vi "Combine_Anomaly_Detection_Results.vi"(4 "Infrnc Dims":cluster{"X Resolution":i32, "Y Resolution":i32}={"X Resolution"=224, "Y Resolution"=224}, 5 "Pixel Results":T1={"Scores(Good)"={"Min"=4.5729, "Max"=58.2981}, "Scores(Bad)"={"Min"=22.3012, "Max"=57.8689}, "F1_Max"=0.3453, "Thrshld(F1_Max)"=38.5075, "IoU_Max"=0.2087, "Thrshld(IoU_Max)"=38.5075, "AUROC"=0.9874, "Prec.(F1_Max)"=0.3041, "Recall(F1_Max)"=0.3994, "FPR(F1_Max)"=0.6006, "FNR(F1_Max)"=0.0} {"FPR(F1_Max)" format="%#_5g"; "FNR(F1_Max)" format="%#_5g"; "Scores(Bad)"."Min" format="%#_5g"; "Scores(Good)"."Min" format="%#_5g"}, 6 "Heatmap Config":T3={"ColorMap_Type"=enum."Jet", "Alpha"=0.4, "Heatmap Range"={"Min"=-1.0, "Max"=-1.0}} {"Heatmap Range"."Min" format="%#_5g"}, 7 "Pixel Anomaly Thrshld":sgl=60.0 format="%_4g", 8 "error in":errorcluster, 9 "Anomaly Map":sgl[][](array[numeric]), 10 "Gt File Path":path, 11 "Img File Path":path=path "D:/DNN/MVTec/screw/test/scratch_head/015.png") -> (0 "error out":errorcluster, 2 "Actual Pixel Threshold":sgl=60.0, 3 "Anomaly Detection Rresults":T5={"Image"="remote image 000001EE05A87998", "Ground Truth"="remote image 000001EE05A87DB8", "Predicted Heat Map"="remote image 000001EE05A87F18", "Predicted Mask"="remote image 000001EE05A87FC8", "Segmentation"="remote image 000001EE05A88968"})   [LabVIEW 2020]
uses:
  PatchCore_AddOn/Low_Level/Controls/Anomaly_Detection_Results_Imgs.ctl
  PatchCore_AddOn/API/Controls/Heatmap_Config.ctl
  PatchCore_AddOn/API/Controls/ColorMap.ctl
  PatchCore_AddOn/API/Controls/MinMax.ctl
  PatchCore_AddOn/API/Controls/Eval_Results.ctl
  <vilib>/vision/Image Controls.llb/IMAQ Image.ctl
  <vilib>/vision/NI_Vision_Development_Module.lvlib
  PatchCore_AddOn/PatchCore_AddOn.lvlib
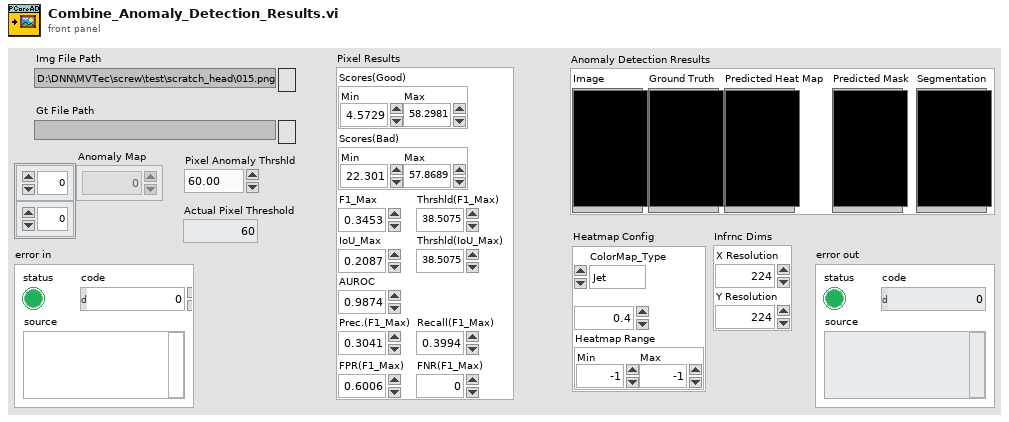
[diagram p1: front panel]
types:
  T1 = typedef "PatchCore_AddOn.lvlib/Eval_Results.ctl" = cluster{"Scores(Good)":T2, "Scores(Bad)":T2, "F1_Max":sgl, "Thrshld(F1_Max)":sgl, "IoU_Max":sgl, "Thrshld(IoU_Max)":sgl, "AUROC":sgl, "Prec.(F1_Max)":sgl, "Recall(F1_Max)":sgl, "FPR(F1_Max)":sgl, "FNR(F1_Max)":sgl}
  T2 = typedef "PatchCore_AddOn.lvlib/MinMax.ctl" = cluster{"Min":sgl, "Max":sgl}
  T3 = typedef "PatchCore_AddOn.lvlib/Heatmap_Config.ctl" = cluster{"ColorMap_Type":T4, "Alpha":sgl, "Heatmap Range":T2}
  T4 = typedef "PatchCore_AddOn.lvlib/ColorMap.ctl" = enum16{"Jet", "Perula", "Inferno", "Plasma", "Viridis"}
  T5 = typedef "PatchCore_AddOn.lvlib/Anomaly_Detection_Results_Imgs.ctl" = cluster{"Image":T6, "Ground Truth":T6, "Predicted Heat Map":T6, "Predicted Mask":T6, "Segmentation":T6}
  T6 = typedef "IMAQ Image.ctl" = refnum<image>
  T7 = typedef "Image Type" = u32
  T8 = cluster{"X Resolution":bool, "Y Resolution":bool}
  T9 = typedef "ROI Descriptor" = cluster{"Global Rectangle":i32[], "Contours":cluster{"ID":enum32{"External", "Internal"}, "Type":u32, "Coordinates":i32[]}[]}
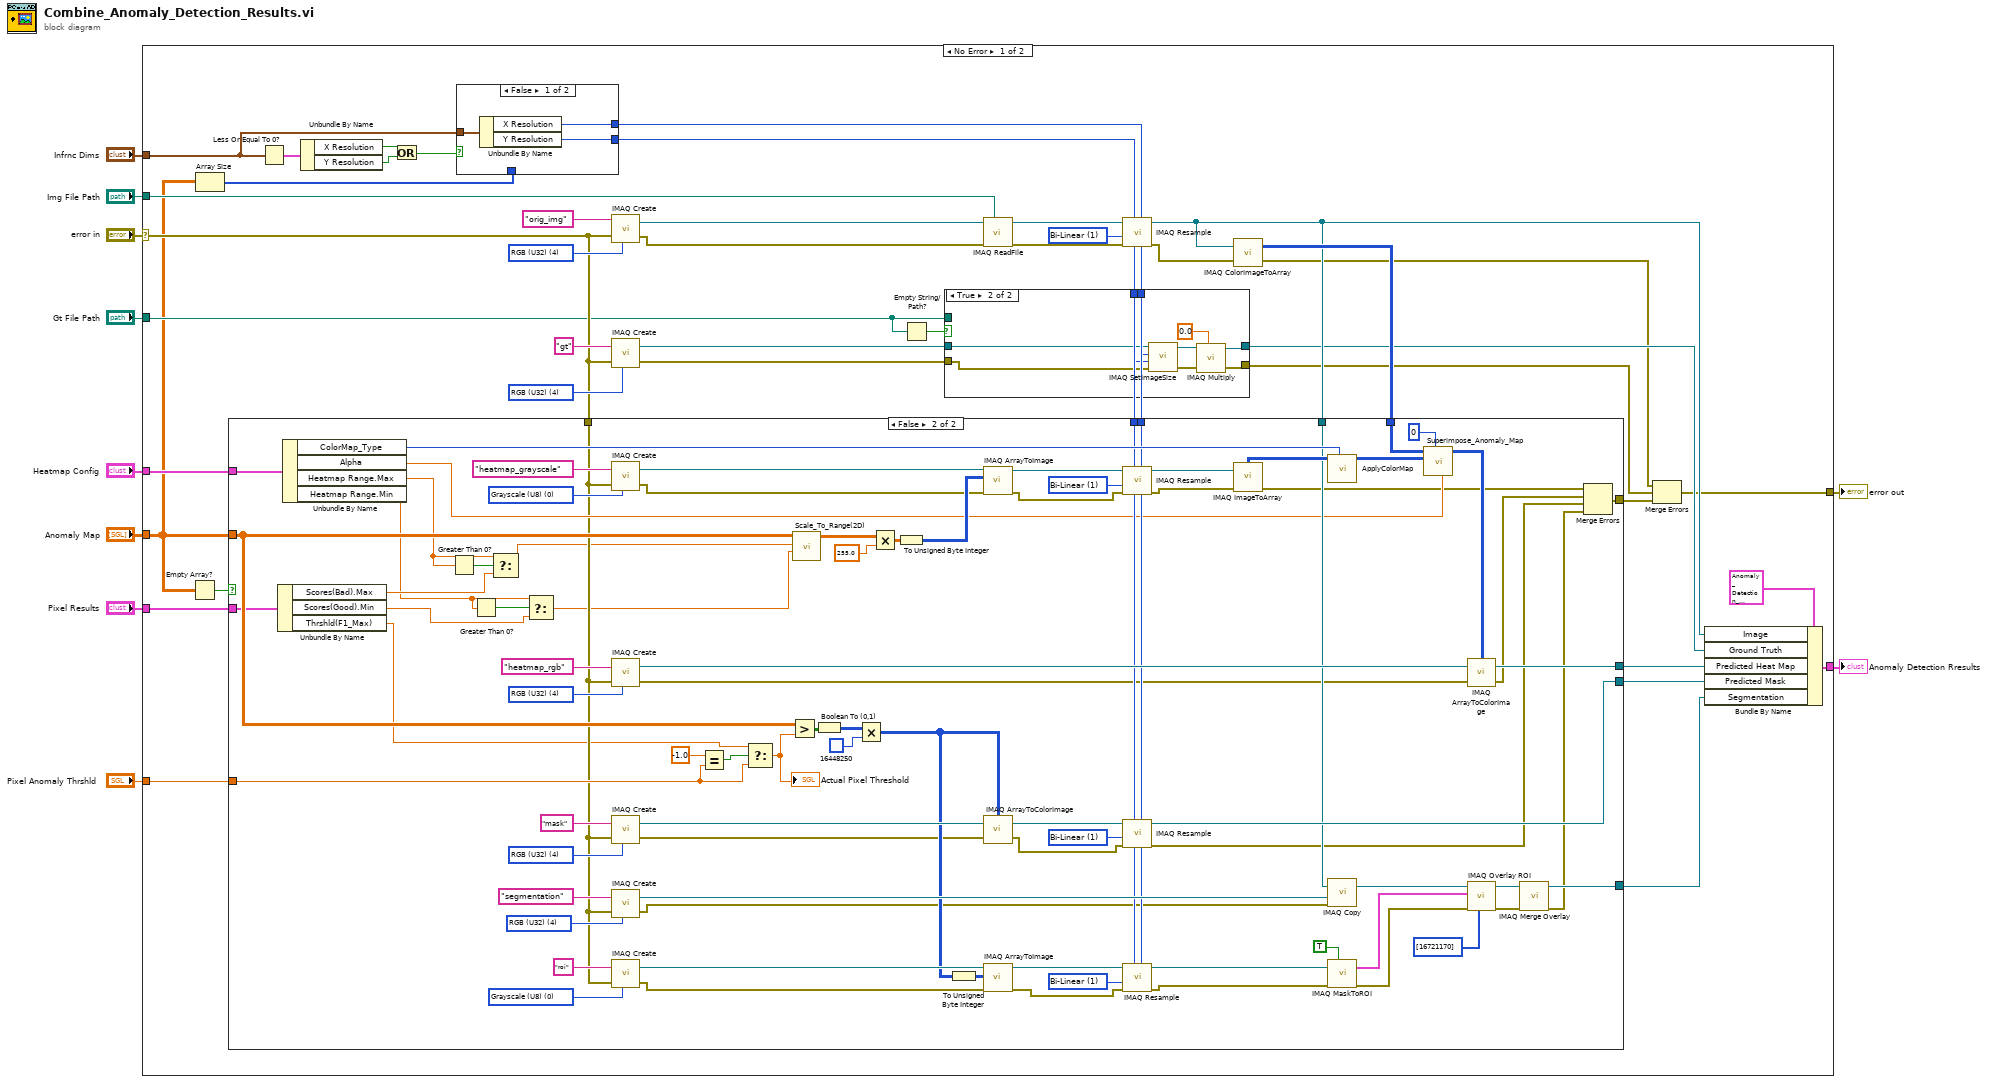
[diagram p0: block diagram]
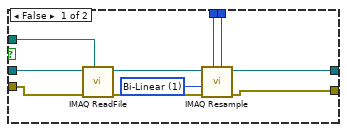
[diagram p3: hidden frame]
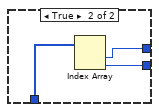
[diagram p4: hidden frame]
diagram:
  n1 = case shown="No Error" "error in" {
    selector: "error in" -> [w19 w162]
    tunnel: [w47 _] -> w10
    tunnel: "Heatmap Config" -> [w43 _]
    tunnel: "Img File Path" -> [w40 _]
    tunnel: "Pixel Anomaly Thrshld" -> [w38 _]
    tunnel: "Infrnc Dims" -> [w29 _]
    tunnel: "Pixel Results" -> [w27 _]
    tunnel: "Gt File Path" -> [w18 _]
    tunnel: [w13 w162] -> w2
    tunnel: "Anomaly Map" -> [w12 _]
    frame No Error {
      w22 = u32 1 items=["Zero Order", "Bi-Linear", "Quadratic", "Cubic Spline"] ("Interpolation Type")
      w39 = T7 4 items=["Grayscale (U8)", "Grayscale (I16)", "Grayscale (SGL)", "Complex (CSG)", "RGB (U32)", "HSL (U32)", "RGB (U64)", "Grayscale (U16)"] ("Image Type")
      w50 = T7 4 items=["Grayscale (U8)", "Grayscale (I16)", "Grayscale (SGL)", "Complex (CSG)", "RGB (U32)", "HSL (U32)", "RGB (U64)", "Grayscale (U16)"] ("Image Type")
      n2 = Empty Array?(array=w12) -> (empty?=w11:bool)
      n3 = Array Size(array=w12) -> (size(s)=w28:i32[])
      n4 = Less Or Equal To 0?(x=w29) -> (x <= 0?=w33:T8)
      n5 = Unbundle By Name(w33) -> ("X Resolution"=w32:bool, "Y Resolution"=w31:bool)
      n6 = Or(x=w32, y=w31) -> (x .or. y?=w30:bool)
      n7 = case shown="False" w30 {
        tunnel: w29 -> [w158 _]
        tunnel: [w157 w160] -> w24
        tunnel: [w156 w159] -> w23
        tunnel: w28 -> [_ w161]
        frame False {
          n8 = Unbundle By Name(w158) -> ("X Resolution"=w157:i32, "Y Resolution"=w156:i32)
        }
        frame True {
          n9 = Index Array(array=w161) -> (element #1=w160:i32, element #2=w159:i32)  [unwired: 2 in]
        }
      }
      n10 = call "IMAQ Create"("Image Name"="orig_img", "Image Type"=w39, "error in (no error)"=w19) -> ("New Image"=w41:T6, "error out"=w20:errorcluster)  [unwired: 2 in]
      n11 = call "IMAQ Create"("Image Name"="gt", "Image Type"=w50, "error in (no error)"=w19) -> ("New Image"=w25:T6, "error out"=w17:errorcluster)  [unwired: 2 in]
      n12 = Empty String/Path?(string/path=w18) -> (empty?=w26:bool)
      n13 = case shown="True" w26 {
        tunnel: w25 -> [w146 w155]
        tunnel: w18 -> [w145 _]
        tunnel: [w144 w149] -> w34
        tunnel: [w142 w148] -> w15
        tunnel: w24 -> [w140 w154]
        tunnel: w23 -> [w139 w153]
        tunnel: w17 -> [w137 w147]
        frame False {
          w138 = u32 1 items=["Zero Order", "Bi-Linear", "Quadratic", "Cubic Spline"] ("Interpolation Type")
          n14 = call "IMAQ ReadFile"("File Path"=w145, "error in (no error)"=w137, "Image"=w146) -> ("error out"=w143:errorcluster, "Image Out"=w141:T6)  [unwired: 4 in, 3 out]
          n15 = call "IMAQ Resample"("X Resolution"=w140, "Y Resolution"=w139, "error in (no error)"=w143, "Interpolation Type"=w138, "Image Src"=w141) -> ("error out"=w142:errorcluster, "Image Dst Out"=w144:T6)  [unwired: 5 in]
        }
        frame True {
          n16 = call "IMAQ SetImageSize"("error in (no error)"=w147, "Y Resolution"=w153, "X Resolution"=w154, "Image"=w155) -> ("error out"=w152:errorcluster, "Image Out"=w151:T6)  [unwired: 1 in]
          n17 = call "IMAQ Multiply"("Image Src A"=w151, "Constant"=0.0, "error in (no error)"=w152) -> ("Image Dst Out"=w149:T6, "error out"=w148:errorcluster)  [unwired: 4 in]
        }
      }
      n18 = call "IMAQ ReadFile"("File Path"=w40, "error in (no error)"=w20, "Image"=w41) -> ("error out"=w35:errorcluster, "Image Out"=w36:T6)  [unwired: 4 in, 3 out]
      n19 = call "IMAQ Resample"("X Resolution"=w24, "Y Resolution"=w23, "error in (no error)"=w35, "Interpolation Type"=w22, "Image Src"=w36) -> ("error out"=w21:errorcluster, "Image Dst Out"=w37:T6)  [unwired: 5 in]
      n20 = call "IMAQ ColorImageToArray"("Image"=w37, "error in (no error)"=w21) -> ("Image Pixels (U32)"=w48:u32[][], "error out"=w16:errorcluster)  [unwired: 2 in, 1 out]
      n21 = case shown="False" w11 {
        tunnel: w48 -> [_ w119]
        tunnel: [_ w107] -> w46
        tunnel: [_ w105] -> w45
        tunnel: [_ w104] -> w44
        tunnel: w43 -> [_ w90]
        tunnel: w38 -> [_ w88]
        tunnel: w37 -> [_ w84]
        tunnel: w12 -> [_ w81]
        tunnel: w27 -> [_ w80]
        tunnel: w24 -> [_ w78]
        tunnel: w23 -> [_ w77]
        tunnel: w19 -> [w52 w74]
        tunnel: [w52 w62] -> w14
        frame True {
        }
        frame False {
          w82 = u32 1 items=["Zero Order", "Bi-Linear", "Quadratic", "Cubic Spline"] ("Interpolation Type")
          w96 = u32 1 items=["Zero Order", "Bi-Linear", "Quadratic", "Cubic Spline"] ("Interpolation Type")
          w100 = T7 0 items=["Grayscale (U8)", "Grayscale (I16)", "Grayscale (SGL)", "Complex (CSG)", "RGB (U32)", "HSL (U32)", "RGB (U64)", "Grayscale (U16)"] ("Image Type")
          w112 = u32 1 items=["Zero Order", "Bi-Linear", "Quadratic", "Cubic Spline"] ("Interpolation Type")
          w117 = T7 4 items=["Grayscale (U8)", "Grayscale (I16)", "Grayscale (SGL)", "Complex (CSG)", "RGB (U32)", "HSL (U32)", "RGB (U64)", "Grayscale (U16)"] ("Image Type")
          w122 = T7 4 items=["Grayscale (U8)", "Grayscale (I16)", "Grayscale (SGL)", "Complex (CSG)", "RGB (U32)", "HSL (U32)", "RGB (U64)", "Grayscale (U16)"] ("Image Type")
          w125 = T7 4 items=["Grayscale (U8)", "Grayscale (I16)", "Grayscale (SGL)", "Complex (CSG)", "RGB (U32)", "HSL (U32)", "RGB (U64)", "Grayscale (U16)"] ("Image Type")
          w135 = T7 0 items=["Grayscale (U8)", "Grayscale (I16)", "Grayscale (SGL)", "Complex (CSG)", "RGB (U32)", "HSL (U32)", "RGB (U64)", "Grayscale (U16)"] ("Image Type")
          n22 = Unbundle By Name(w80) -> ("Scores(Bad).Max"=w60:sgl, "Scores(Good).Min"=w57:sgl, "Thrshld(F1_Max)"=w55:sgl)
          n23 = Unbundle By Name(w90) -> ("ColorMap_Type"=w89:T4, "Alpha"=w76:sgl, "Heatmap Range.Max"=w53:sgl, "Heatmap Range.Min"=w54:sgl)
          n24 = Greater Than 0?(x=w53) -> (x > 0?=w59:bool)
          n25 = Greater Than 0?(x=w54) -> (x > 0?=w56:bool)
          n26 = Select(t=w53, s=w59, f=w60) -> (s? t:f=w61:sgl)
          n27 = Select(t=w54, s=w56, f=w57) -> (s? t:f=w58:sgl)
          n28 = call "IMAQ Create"("Image Name"="heatmap_grayscale", "Image Type"=w100, "error in (no error)"=w74) -> ("New Image"=w99:T6, "error out"=w72:errorcluster)  [unwired: 2 in]
          n29 = call "IMAQ Create"("Image Name"="heatmap_rgb", "Image Type"=w125, "error in (no error)"=w74) -> ("New Image"=w124:T6, "error out"=w67:errorcluster)  [unwired: 2 in]
          n30 = call "IMAQ Create"("Image Name"="mask", "Image Type"=w122, "error in (no error)"=w74) -> ("New Image"=w120:T6, "error out"=w75:errorcluster)  [unwired: 2 in]
          n31 = call "IMAQ Create"("Image Name"="segmentation", "Image Type"=w117, "error in (no error)"=w74) -> ("New Image"=w115:T6, "error out"=w68:errorcluster)  [unwired: 2 in]
          n32 = call "IMAQ Create"("Image Name"="roi", "Image Type"=w135, "error in (no error)"=w74) -> ("New Image"=w134:T6, "error out"=w69:errorcluster)  [unwired: 2 in]
          n33 = Equal?(x=sgl -1.0 ("y"), y=w88) -> (x = y?=w87:bool)
          n34 = Select(t=w55, s=w87, f=w88) -> (s? t:f=w79:sgl)
          "Actual Pixel Threshold" <- w79
          n35 = Greater?(x=w81, y=w79) -> (0:w130:bool[][])
          n36 = call "Scale_To_Range(2D).vi"("min pixel score"=w58, "max pixel score"=w61, "anomaly map"=w81) -> ("anomaly map normalized"=w133:sgl[][])  [unwired: 8 in]
          n37 = Boolean To (0,1)(Boolean=w130) -> (0, 1=w131:i16[][])
          n38 = Multiply(x=w131, y=u32 16448250) -> (x*y=w114:u32[][])
          n39 = Multiply(x=w133, y=sgl 255.0) -> (x*y=w103:sgl[][])
          n40 = To Unsigned Byte Integer(number=w103) -> (unsigned 8bit integer=w102:u8[][])
          n41 = To Unsigned Byte Integer(number=w114) -> (unsigned 8bit integer=w109:u8[][])
          n42 = call "IMAQ ArrayToImage"("error in (no error)"=w72, "Image Pixels (U8)"=w102, "Image"=w99) -> ("error out"=w73:errorcluster, "Image Out"=w98:T6)  [unwired: 7 in]
          n43 = call "IMAQ ArrayToColorImage"("Image Pixels (U32)"=w114, "Image"=w120, "error in (no error)"=w75) -> ("Image Out"=w111:T6, "error out"=w71:errorcluster)  [unwired: 2 in]
          n44 = call "IMAQ ArrayToImage"("error in (no error)"=w69, "Image Pixels (U8)"=w109, "Image"=w134) -> ("error out"=w70:errorcluster, "Image Out"=w92:T6)  [unwired: 7 in]
          n45 = call "IMAQ Resample"("X Resolution"=w78, "Y Resolution"=w77, "error in (no error)"=w73, "Interpolation Type"=w96, "Image Src"=w98) -> ("error out"=w95:errorcluster, "Image Dst Out"=w97:T6)  [unwired: 5 in]
          n46 = call "IMAQ Resample"("X Resolution"=w78, "Y Resolution"=w77, "error in (no error)"=w71, "Interpolation Type"=w112, "Image Src"=w111) -> ("error out"=w65:errorcluster, "Image Dst Out"=w104:T6)  [unwired: 5 in]
          n47 = call "IMAQ Resample"("X Resolution"=w78, "Y Resolution"=w77, "error in (no error)"=w70, "Interpolation Type"=w82, "Image Src"=w92) -> ("error out"=w91:errorcluster, "Image Dst Out"=w93:T6)  [unwired: 5 in]
          n48 = call "IMAQ ImageToArray"("error in (no error)"=w95, "Image"=w97) -> ("error out"=w63:errorcluster, "Image Pixels (U8)"=w94:u8[][])  [unwired: 2 in, 3 out]
          n49 = call "ApplyColorMap.vi"("ColorMap Type"=w89, "Image in"=w94) -> ("Image out"=w113:u32[][])  [unwired: 9 in]
          n50 = call "IMAQ Copy"("error in (no error)"=w68, "Image Dst"=w115, "Image Src"=w84) -> ("Image Dst Out"=w118:T6)  [unwired: 3 in, 1 out]
          n51 = call "IMAQ MaskToROI"("External edges only (T)"=TRUE, "Image"=w93, "error in (no error)"=w91) -> ("ROI Descriptor"=w83:T9, "error out"=w85:errorcluster)  [unwired: 4 in, 1 out]
          n52 = call "Superimpose_Anomaly_Map.vi"("Alpha"=w76, "Gamma"=0, "Anomaly Map"=w113, "Image"=w119) -> ("Img out"=w127:u32[][])  [unwired: 7 in]
          n53 = call "IMAQ ArrayToColorImage"("Image Pixels (U32)"=w127, "Image"=w124, "error in (no error)"=w67) -> ("Image Out"=w105:T6, "error out"=w64:errorcluster)  [unwired: 2 in]
          n54 = call "IMAQ Overlay ROI"("Colors (Green)"=u32[] [16721170], "error in (no error)"=w85, "ROI Descriptor"=w83, "Image"=w118) -> ("error out"=w106:errorcluster, "Image Out"=w108:T6)  [unwired: 6 in]
          n55 = call "IMAQ Merge Overlay"("error in (no error)"=w106, "Image Src"=w108) -> ("error out"=w66:errorcluster, "Image Dst Out"=w107:T6)  [unwired: 8 in]
          n56 = Merge Errors(w63, w64, w65, w66) -> (w62:errorcluster)
        }
      }
      n57 = Merge Errors(w16, w15, w14) -> (w13:errorcluster)
      n58 = Bundle By Name(cluster=T5 {"Image"=refnum, "Ground Truth"=refnum, "Predicted Heat Map"=refnum, "Predicted Mask"=refnum, "Segmentation"=refnum} ("Anomaly Detection Results"), "Image"=w37, "Ground Truth"=w34, "Predicted Heat Map"=w45, "Predicted Mask"=w44, "Segmentation"=w46) -> (w47:T5)
    }
    frame Error {
    }
  }
  "error out" <- w2
  "Anomaly Detection Rresults" <- w10
